vi "VMI_create_image_from_points_new.vi"(0 "Centroid?":bool, 2 "New Array":bool, 3 "Image Info":T1={"X size"=782.0, "Y size"=582.0, "Centroiding"=1.0}, 4 "Input array":i16[][](array[numeric]), 5 "Points":cluster{"X":sgl, "Y":sgl}[](array[cluster])=array[24000 elements]) -> (1 "Image Array":i16[][](array[numeric]))   [LabVIEW 2020]
uses:
  Type defs/Image_info.ctl
panel:
  out "Intensity Graph 2":i16[][](graph)
  out "sum":i32
  out "Numeric":i32
  out "size(s)":i32
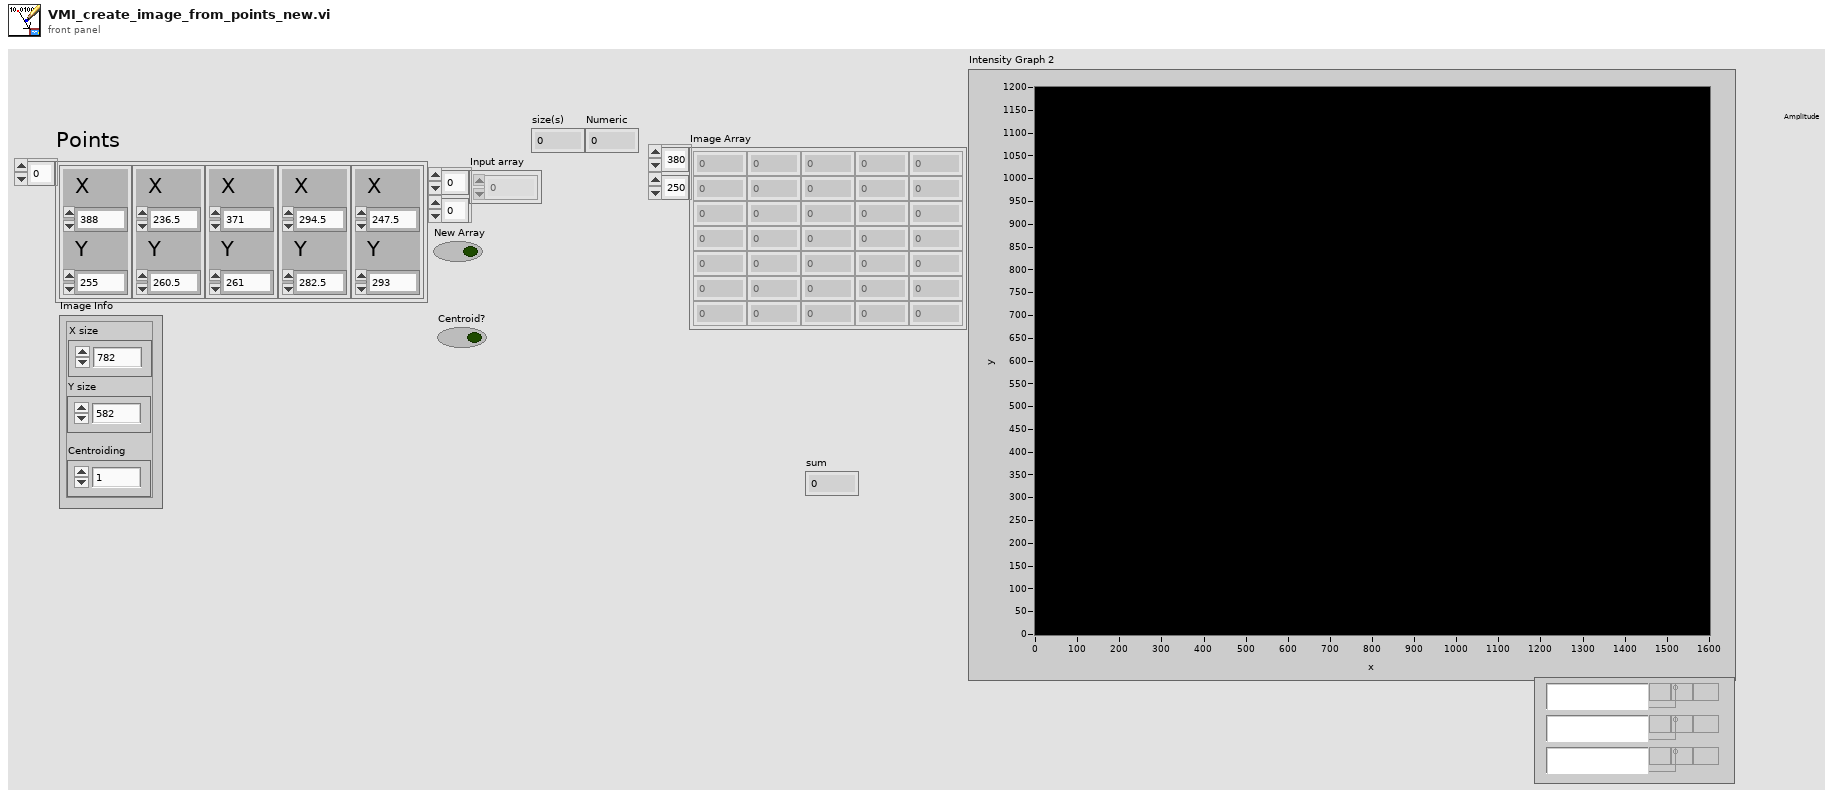
[diagram p1: front panel]
types:
  T1 = typedef "Image_info.ctl" = cluster{"X size":dbl, "Y size":dbl, "Centroiding":dbl}
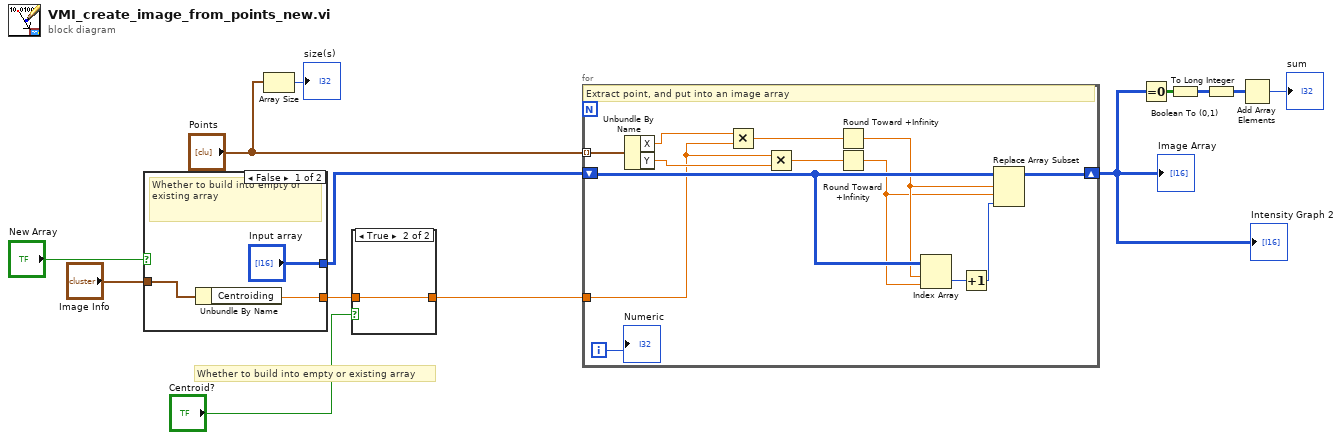
[diagram p0: block diagram]
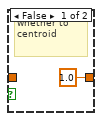
[diagram p2: hidden frame]
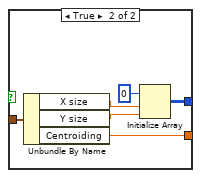
[diagram p3: hidden frame]
diagram:
  # "Whether to build into empty or existing array"
  n1 = case shown="False" "New Array" {
    tunnel: "Image Info" -> [w15 w21]
    tunnel: ["Input array" w18] -> w7
    tunnel: [w14 w17] -> w2
    frame False {
      # "Whether to build into empty or existing array"
      n2 = Unbundle By Name(w15) -> ("Centroiding"=w14:dbl)
    }
    frame True {
      n3 = Unbundle By Name(w21) -> ("X size"=w20:dbl, "Y size"=w19:dbl, "Centroiding"=w17:dbl)
      n4 = Initialize Array(i16 0 ("element"), w20, w19) -> (w18:i16[][])
    }
  }
  n5 = Array Size(array="Points") -> (size(s)=→"size(s)":i32)
  n6 = case shown="True" "Centroid?" {
    tunnel: [1.0 ("Centroiding") w24] -> w3
    tunnel: w2 -> [_ w24]
    frame False {
      # "whether to centroid"
    }
    frame True {
    }
  }
  n7 = for {
    tunnel: "Points" -> [w37] mode=indexing
    shift-right: [w34] -> w4
    shift-left: w7 -> [w32]
    tunnel: w3 -> [w25]
    i -> [w33]
    # "Extract point, and put into an image array"
    n8 = Unbundle By Name(w37) -> ("X"=w28:sgl, "Y"=w26:sgl)
    n9 = Multiply(x=w28, y=w25) -> (x*y=w29:dbl)
    n10 = Multiply(x=w25, y=w26) -> (x*y=w27:dbl)
    n11 = Round Toward +Infinity(x=w29) -> (ceil(x): smallest int >= x=w31:dbl)
    n12 = Round Toward +Infinity(x=w27) -> (ceil(x): smallest int >= x=w30:dbl)
    n13 = Index Array(array=w32, index (row)=w31, index (col)=w30) -> (element=w36:i16)
    n14 = Increment(x=w36) -> (x+1=w35:i16)
    n15 = Replace Array Subset(array=w32, new element=w35, index (row)=w31, index (col)=w30) -> (w34:i16[][])
    "Numeric" <- w33
  }
  "Image Array" <- w4
  "Intensity Graph 2" <- w4
  n16 = Equal To 0?(x=w4) -> (x = 0?=w11:bool[][])
  n17 = Boolean To (0,1)(Boolean=w11) -> (0, 1=w10:i16[][])
  n18 = To Long Integer(number=w10) -> (32bit integer=w9:i32[][])
  n19 = Add Array Elements(numeric array=w9) -> (sum=→"sum":i32)
